vi "NMEA_Paser.vi"(8 "error in":errorcluster, 10 "INPUT":string) -> (0 "error out":errorcluster, 2 "output":string)   [LabVIEW 2015]
panel:
  # ","
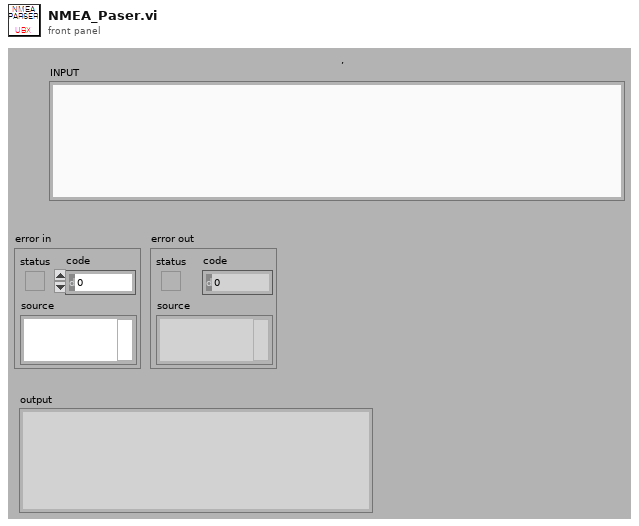
[diagram p1: front panel]
types:
  T1 = cluster{"UTC":dbl, "N/S":i8, "Latitude":dbl, "N/S 2":i8, "Longitude":dbl, "N/S 3":i8, "Speed over ground":dbl, "Course over ground":dbl}
  T2 = cluster{"UTC":dbl, "Latitude 3":dbl, "N/S":u8, "Longitude 3":dbl, "Longitude 4":dbl, "Longitude 5":dbl, "Longitude 6":dbl}
  T3 = enum16{"None", "APB", "BOD", "GGA", "GLL", "GSA", "GSV", "RMB", "RMC", "RTE", "WPL", "APA", "VTG", "XTE"}
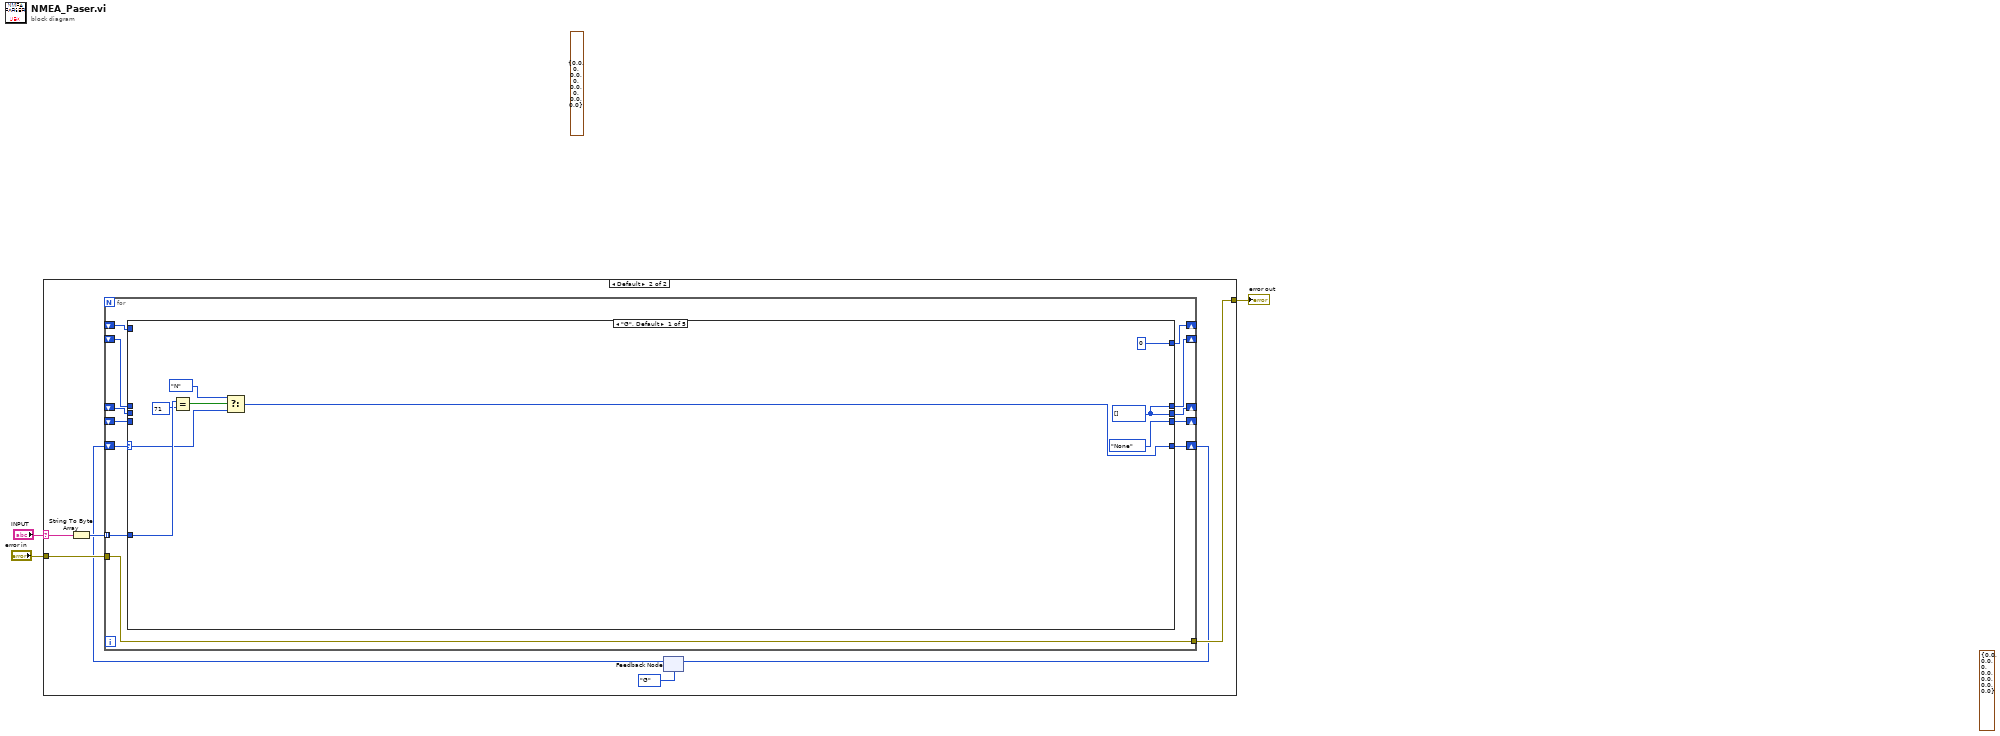
[diagram p0: block diagram]
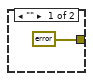
[diagram p2: hidden frame]
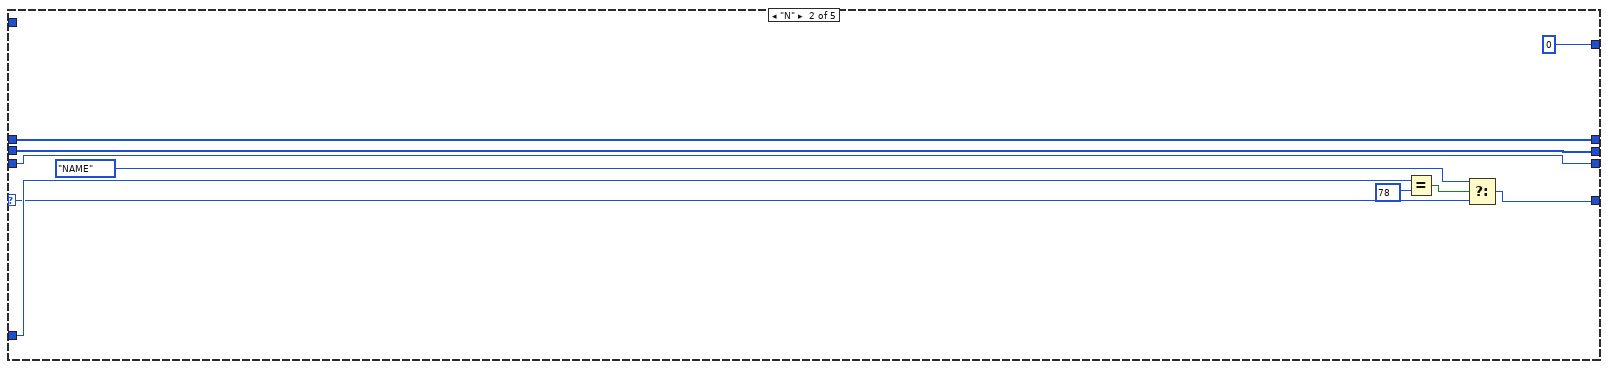
[diagram p3: hidden frame]
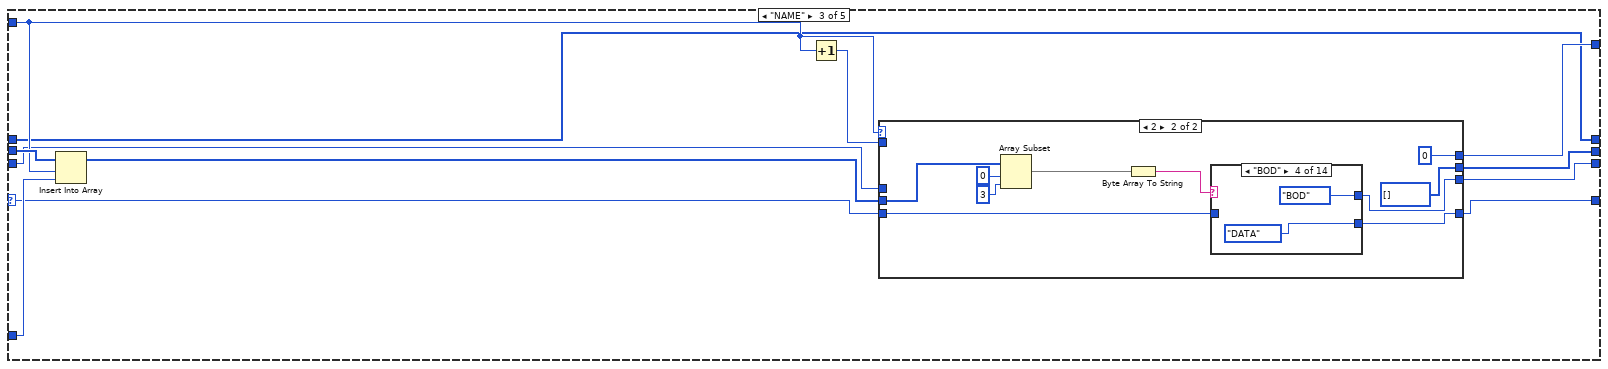
[diagram p4: hidden frame]
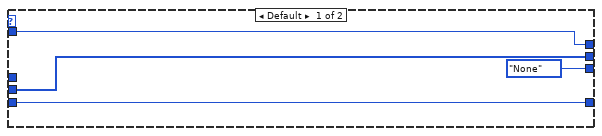
[diagram p5: hidden frame]
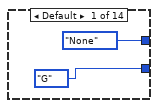
[diagram p6: hidden frame]
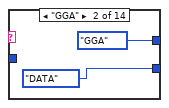
[diagram p7: hidden frame]
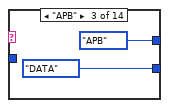
[diagram p8: hidden frame]
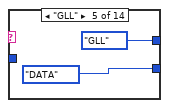
[diagram p9: hidden frame]
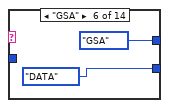
[diagram p10: hidden frame]
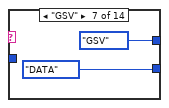
[diagram p11: hidden frame]
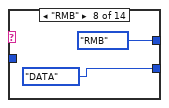
[diagram p12: hidden frame]
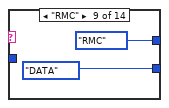
[diagram p13: hidden frame]
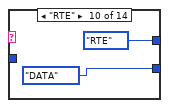
[diagram p14: hidden frame]
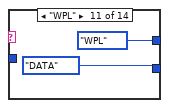
[diagram p15: hidden frame]
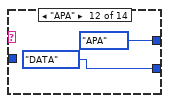
[diagram p16: hidden frame]
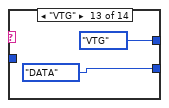
[diagram p17: hidden frame]
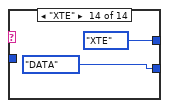
[diagram p18: hidden frame]
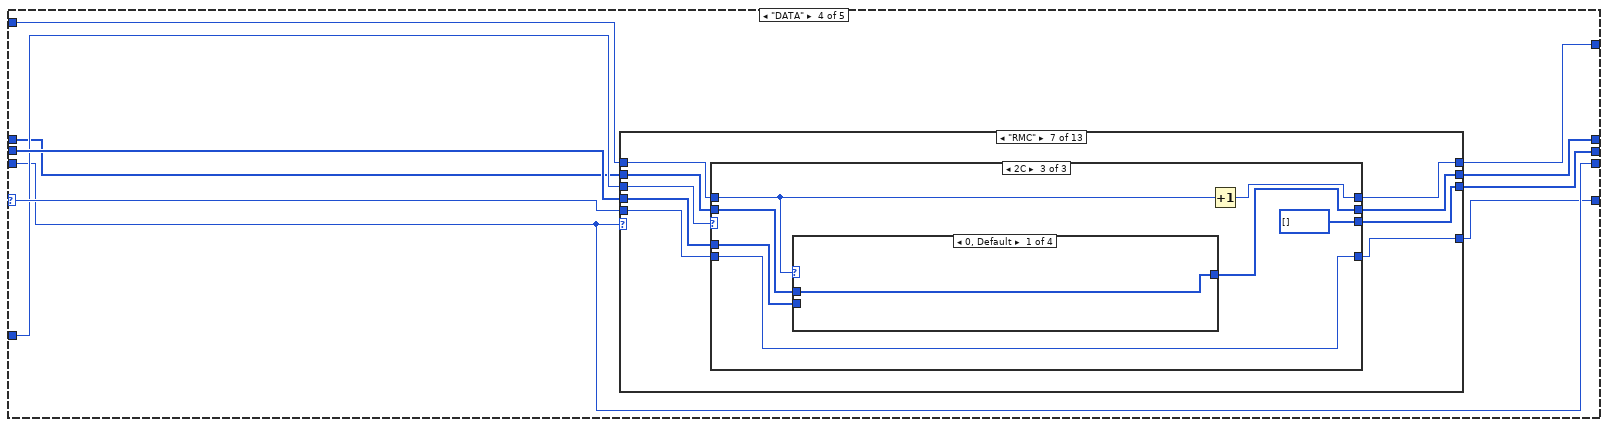
[diagram p19: hidden frame]
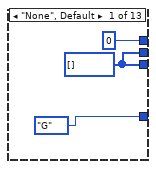
[diagram p20: hidden frame]
diagram:
  (unwired) T1 {"UTC"=0.0, "N/S"=0, "Latitude"=0.0, "N/S 2"=0, "Longitude"=0.0, "N/S 3"=0, "Speed over ground"=0.0, "Course over ground"=0.0} ("클러스터")
  (unwired) T2 {"UTC"=0.0, "Latitude 3"=0.0, "N/S"=0, "Longitude 3"=0.0, "Longitude 4"=0.0, "Longitude 5"=0.0, "Longitude 6"=0.0} ("클러스터 2")
  n1 = case shown="Default" "INPUT" {
    selector: "INPUT" -> [_ w8]
    tunnel: "error in" -> [_ w10]
    tunnel: [errorcluster {"status"=TRUE, "code"=0, "source"="Input Data is blank"} ("error in") w9] -> w2
    frame "" {
    }
    frame Default {
      n2 = String To Byte Array(string=w8) -> (unsigned byte array=w11:u8[])
      n3 = feedback #1(enum16{"G", "N", "NAME", "DATA", "END"}."G" ("t")) -> (w5:enum16{"G", "N", "NAME", "DATA", "END"})
      n4 = for {
        tunnel: w11 -> [w23] mode=indexing
        shift-right: [w22] -> _
        shift-left: _ -> [w19]
        shift-right: [w21] -> _
        shift-left: _ -> [w20]
        shift-right: [w18] -> _
        shift-left: _ -> [w17]
        shift-right: [w16] -> _
        shift-left: _ -> [w15]
        tunnel: w10 -> [w14]
        tunnel: [w14] -> w9
        shift-right: [w12] -> w6
        shift-left: w5 -> [w13]
        n5 = case shown="\"G\", Default" w13 {
          selector: w13 -> [w26 w34 w51 w105 _]
          tunnel: w23 -> [w32 w42 w53 w104 w576]
          tunnel: [0 0 w48 w99 w582] -> w22
          tunnel: [w27 w39 w44 w102 w581] -> w21
          tunnel: w20 -> [_ w39 w54 w106 w572]
          tunnel: w19 -> [_ _ w50 w101 w571]
          tunnel: [T3."None" w38 w47 w103 w583] -> w18
          tunnel: w17 -> [_ w38 w46 w103 w580]
          tunnel: [w27 w37 w45 w98 w570] -> w16
          tunnel: w15 -> [_ w37 w45 w100 w579]
          tunnel: [w24 w33 w43 w97 w569] -> w12
          frame "G", Default {
            w27 = u8[] []
            n6 = Equal?(x=w32, y=u8 71) -> (x = y?=w30:bool)
            n7 = Select(t=enum16{"G", "N", "NAME", "DATA", "END"}."N", s=w30, f=w26) -> (s? t:f=w24:enum16{"G", "N", "NAME", "DATA", "END"})
          }
          frame "N" {
            n8 = Equal?(x=w42, y=u8 78) -> (x = y?=w36:bool)
            n9 = Select(t=enum16{"G", "N", "NAME", "DATA", "END"}."NAME", s=w36, f=w34) -> (s? t:f=w33:enum16{"G", "N", "NAME", "DATA", "END"})
          }
          frame "NAME" {
            n10 = Insert Into Array(array=w54, index=w50, new element=w53) -> (w52:u8[])
            n11 = Increment(x=w50) -> (x+1=w49:i32)
            n12 = case shown="2" w50 {
              tunnel: w52 -> [w55 w61]
              tunnel: w51 -> [w58 w64]
              tunnel: [w58 w59] -> w43
              tunnel: [w57 0] -> w48
              tunnel: w49 -> [w57 _]
              tunnel: [T3."None" w62] -> w47
              tunnel: w46 -> [_ _]
              tunnel: [w55 u8[] []] -> w44
              frame Default {
              }
              frame 2 {
                n13 = Array Subset(array=w61, index=0, length=3) -> (w66:u8[])
                n14 = Byte Array To String(unsigned byte array=w66) -> (string=w65:string)
                n15 = case shown="\"BOD\"" w65 {
                  tunnel: w64 -> [_ _ _ _ _ _ _ _ _ _ _ _ _ _]
                  tunnel: [T3."None" T3."GGA" T3."APB" T3."BOD" T3."GLL" T3."GSA" T3."GSV" T3."RMB" T3."RMC" T3."RTE" T3."WPL" T3."APA" T3."VTG" T3."XTE"] -> w62
                  tunnel: [enum16{"G", "N", "NAME", "DATA", "END"}."G" ("t") enum16{"G", "N", "NAME", "DATA", "END"}."DATA" ("t") enum16{"G", "N", "NAME", "DATA", "END"}."DATA" ("t") enum16{"G", "N", "NAME", "DATA", "END"}."DATA" ("t") enum16{"G", "N", "NAME", "DATA", "END"}."DATA" ("t") enum16{"G", "N", "NAME", "DATA", "END"}."DATA" ("t") enum16{"G", "N", "NAME", "DATA", "END"}."DATA" ("t") enum16{"G", "N", "NAME", "DATA", "END"}."DATA" ("t") enum16{"G", "N", "NAME", "DATA", "END"}."DATA" ("t") enum16{"G", "N", "NAME", "DATA", "END"}."DATA" ("t") enum16{"G", "N", "NAME", "DATA", "END"}."DATA" ("t") enum16{"G", "N", "NAME", "DATA", "END"}."DATA" ("t") enum16{"G", "N", "NAME", "DATA", "END"}."DATA" ("t") enum16{"G", "N", "NAME", "DATA", "END"}."DATA" ("t")] -> w59
                  frame Default {
                  }
                  frame "GGA" {
                  }
                  frame "APB" {
                  }
                  frame "BOD" {
                  }
                  frame "GLL" {
                  }
                  frame "GSA" {
                  }
                  frame "GSV" {
                  }
                  frame "RMB" {
                  }
                  frame "RMC" {
                  }
                  frame "RTE" {
                  }
                  frame "WPL" {
                  }
                  frame "APA" {
                  }
                  frame "VTG" {
                  }
                  frame "XTE" {
                  }
                }
              }
            }
          }
          frame "DATA" {
            n16 = case shown="\"RMC\"" w103 {
              tunnel: w104 -> [_ w118 w160 w202 w238 w280 w322 w364 w400 w436 w472 w508 w541]
              tunnel: w106 -> [_ w116 w158 w200 w236 w278 w320 w362 w398 w434 w470 w506 w539]
              tunnel: w105 -> [_ w117 w159 w201 w237 w279 w321 w363 w399 w435 w471 w507 w540]
              tunnel: [w108 w115 w157 w199 w235 w277 w319 w361 w397 w433 w469 w505 w538] -> w102
              tunnel: w101 -> [_ w114 w156 w198 w234 w276 w318 w360 w396 w432 w468 w504 w537]
              tunnel: w100 -> [_ w113 w155 w197 w233 w275 w317 w359 w395 w431 w467 w503 w536]
              tunnel: [w108 w112 w154 w196 w232 w274 w316 w358 w394 w430 w466 w502 w535] -> w98
              tunnel: [0 w111 w153 w195 w231 w273 w315 w357 w393 w429 w465 w501 w534] -> w99
              tunnel: [enum16{"G", "N", "NAME", "DATA", "END"}."G" ("t") w110 w152 w194 w230 w272 w314 w356 w392 w428 w464 w500 w533] -> w97
              frame "None", Default {
                w108 = u8[] []
              }
              frame "APB" {
                n17 = case shown="Default" w118 {
                  selector: w118 -> [w123 _ _]
                  tunnel: [w121 enum16{"G", "N", "NAME", "DATA", "END"}."END" ("t") w135] -> w110
                  tunnel: w117 -> [w121 _ w135]
                  tunnel: w116 -> [w124 _ w133]
                  tunnel: [w122 u8[] [] u8[] []] -> w115
                  tunnel: w114 -> [w119 _ w129]
                  tunnel: w113 -> [w120 w126 w132]
                  tunnel: [w120 w126 w131] -> w112
                  tunnel: [w119 0 w130] -> w111
                  frame Default {
                    n18 = Insert Into Array(array=w124, new element=w123) -> (w122:u8[])  [unwired: 1 in]
                  }
                  frame 42 {
                  }
                  frame 44 {
                    n19 = case shown="1, 2, 4..7, 9, 10, 12, 14" w129 {
                      tunnel: w133 -> [_ w138 w141 w149]
                      tunnel: w132 -> [w136 w139 w145 w147]
                      tunnel: [w136 w137 w144 w151] -> w131
                      frame 0, Default {
                      }
                      frame 1, 2, 4..7, 9, 10, 12, 14 {
                        n20 = Insert Into Array(array=w139, new element=w138) -> (w137:u8[])  [unwired: 1 in]
                      }
                      frame 3 {
                        n21 = Byte Array To String(unsigned byte array=w141) -> (string=w143:string)
                        n22 = Fract/Exp String To Number(string=w143) -> (number=w142:dbl)  [unwired: 3 in, 1 out]
                        n23 = Type Cast(type=w141, x=w142) -> (*(type *) &x=w140:u8[])
                        n24 = Insert Into Array(array=w145, new element=w140) -> (w144:u8[])  [unwired: 1 in]
                      }
                      frame 8, 11 {
                        n25 = Byte Array To String(unsigned byte array=w149) -> (string=w150:string)
                        n26 = Decimal String To Number(string=w150) -> (number=w148:i32)  [unwired: 2 in, 1 out]
                        n27 = Type Cast(type=w147, x=w148) -> (*(type *) &x=w146:u8[])
                        n28 = Insert Into Array(array=w147, new element=w146) -> (w151:u8[])  [unwired: 1 in]
                      }
                    }
                    n29 = Increment(x=w129) -> (x+1=w130:i32)
                  }
                }
              }
              frame "GGA" {
                n30 = case shown="2C" w160 {
                  selector: w160 -> [w165 _ _]
                  tunnel: [w163 enum16{"G", "N", "NAME", "DATA", "END"}."END" ("t") w177] -> w152
                  tunnel: w159 -> [w163 _ w177]
                  tunnel: w158 -> [w166 _ w171]
                  tunnel: [w164 u8[] [] u8[] []] -> w157
                  tunnel: w156 -> [w161 _ w173]
                  tunnel: w155 -> [w162 w168 w172]
                  tunnel: [w162 w168 w175] -> w154
                  tunnel: [w161 0 w174] -> w153
                  frame Default {
                    n31 = Insert Into Array(array=w166, new element=w165) -> (w164:u8[])  [unwired: 1 in]
                  }
                  frame 42 {
                  }
                  frame 44 {
                    n32 = case shown="3, 5, 10, 12" w173 {
                      tunnel: w171 -> [_ w179 w183 w191]
                      tunnel: w172 -> [w178 w181 w185 w189]
                      tunnel: [w178 w180 w187 w193] -> w175
                      frame 0, Default {
                      }
                      frame 3, 5, 10, 12 {
                        n33 = Insert Into Array(array=w181, new element=w179) -> (w180:u8[])  [unwired: 1 in]
                      }
                      frame 1, 2, 4, 8, 9, 11, 13 {
                        n34 = Byte Array To String(unsigned byte array=w183) -> (string=w186:string)
                        n35 = Fract/Exp String To Number(string=w186) -> (number=w184:dbl)  [unwired: 3 in, 1 out]
                        n36 = Type Cast(type=w183, x=w184) -> (*(type *) &x=w182:u8[])
                        n37 = Insert Into Array(array=w185, new element=w182) -> (w187:u8[])  [unwired: 1 in]
                      }
                      frame 6, 7 {
                        n38 = Byte Array To String(unsigned byte array=w191) -> (string=w192:string)
                        n39 = Decimal String To Number(string=w192) -> (number=w190:i32)  [unwired: 2 in, 1 out]
                        n40 = Type Cast(type=w189, x=w190) -> (*(type *) &x=w188:u8[])
                        n41 = Insert Into Array(array=w189, new element=w188) -> (w193:u8[])  [unwired: 1 in]
                      }
                    }
                    n42 = Increment(x=w173) -> (x+1=w174:i32)
                  }
                }
              }
              frame "GLL" {
                n43 = case shown="Default" w202 {
                  selector: w202 -> [w207 _ _]
                  tunnel: [w205 enum16{"G", "N", "NAME", "DATA", "END"}."END" ("t") w219] -> w194
                  tunnel: w201 -> [w205 _ w219]
                  tunnel: w200 -> [w208 _ w217]
                  tunnel: [w206 u8[] [] u8[] []] -> w199
                  tunnel: w198 -> [w203 _ w213]
                  tunnel: w197 -> [w204 w210 w216]
                  tunnel: [w204 w210 w215] -> w196
                  tunnel: [w203 0 w214] -> w195
                  frame Default {
                    n44 = Insert Into Array(array=w208, new element=w207) -> (w206:u8[])  [unwired: 1 in]
                  }
                  frame 42 {
                  }
                  frame 44 {
                    n45 = case shown="0, Default" w213 {
                      tunnel: w217 -> [_ w222 w225]
                      tunnel: w216 -> [w220 w223 w229]
                      tunnel: [w220 w221 w228] -> w215
                      frame 0, Default {
                      }
                      frame 2, 4, 6 {
                        n46 = Insert Into Array(array=w223, new element=w222) -> (w221:u8[])  [unwired: 1 in]
                      }
                      frame 1, 3, 5 {
                        n47 = Byte Array To String(unsigned byte array=w225) -> (string=w227:string)
                        n48 = Fract/Exp String To Number(string=w227) -> (number=w226:dbl)  [unwired: 3 in, 1 out]
                        n49 = Type Cast(type=w225, x=w226) -> (*(type *) &x=w224:u8[])
                        n50 = Insert Into Array(array=w229, new element=w224) -> (w228:u8[])  [unwired: 1 in]
                      }
                    }
                    n51 = Increment(x=w213) -> (x+1=w214:i32)
                  }
                }
              }
              frame "GSA" {
                n52 = case shown="2A" w238 {
                  selector: w238 -> [w243 _ _]
                  tunnel: [w241 enum16{"G", "N", "NAME", "DATA", "END"}."END" ("t") w255] -> w230
                  tunnel: w237 -> [w241 _ w255]
                  tunnel: w236 -> [w244 _ w253]
                  tunnel: [w242 u8[] [] u8[] []] -> w235
                  tunnel: w234 -> [w239 _ w249]
                  tunnel: w233 -> [w240 w246 w252]
                  tunnel: [w240 w246 w251] -> w232
                  tunnel: [w239 0 w250] -> w231
                  frame Default {
                    n53 = Insert Into Array(array=w244, new element=w243) -> (w242:u8[])  [unwired: 1 in]
                  }
                  frame 42 {
                  }
                  frame 44 {
                    n54 = case shown="3..14" w249 {
                      tunnel: w253 -> [_ w257 w261 w269]
                      tunnel: w252 -> [w256 w258 w265 w267]
                      tunnel: [w256 w259 w264 w271] -> w251
                      frame 0, Default {
                      }
                      frame 1 {
                        n55 = Insert Into Array(array=w258, new element=w257) -> (w259:u8[])  [unwired: 1 in]
                      }
                      frame 15..17 {
                        n56 = Byte Array To String(unsigned byte array=w261) -> (string=w263:string)
                        n57 = Fract/Exp String To Number(string=w263) -> (number=w262:dbl)  [unwired: 3 in, 1 out]
                        n58 = Type Cast(type=w261, x=w262) -> (*(type *) &x=w260:u8[])
                        n59 = Insert Into Array(array=w265, new element=w260) -> (w264:u8[])  [unwired: 1 in]
                      }
                      frame 3..14 {
                        n60 = Byte Array To String(unsigned byte array=w269) -> (string=w270:string)
                        n61 = Decimal String To Number(string=w270) -> (number=w266:i32)  [unwired: 2 in, 1 out]
                        n62 = Type Cast(type=w267, x=w266) -> (*(type *) &x=w268:u8[])
                        n63 = Insert Into Array(array=w267, new element=w268) -> (w271:u8[])  [unwired: 1 in]
                      }
                    }
                    n64 = Increment(x=w249) -> (x+1=w250:i32)
                  }
                }
              }
              frame "RMB" {
                n65 = case shown="2A" w280 {
                  selector: w280 -> [w285 _ _]
                  tunnel: [w283 enum16{"G", "N", "NAME", "DATA", "END"}."END" ("t") w297] -> w272
                  tunnel: w279 -> [w283 _ w297]
                  tunnel: w278 -> [w286 _ w295]
                  tunnel: [w284 u8[] [] u8[] []] -> w277
                  tunnel: w276 -> [w281 _ w291]
                  tunnel: w275 -> [w282 w288 w294]
                  tunnel: [w282 w288 w293] -> w274
                  tunnel: [w281 0 w292] -> w273
                  frame Default {
                    n66 = Insert Into Array(array=w286, new element=w285) -> (w284:u8[])  [unwired: 1 in]
                  }
                  frame 42 {
                  }
                  frame 44 {
                    n67 = case shown="0, Default" w291 {
                      tunnel: w295 -> [_ w300 w303 w311]
                      tunnel: w294 -> [w298 w301 w307 w309]
                      tunnel: [w298 w299 w306 w313] -> w293
                      frame 0, Default {
                      }
                      frame 1, 3, 7, 9, 13 {
                        n68 = Insert Into Array(array=w301, new element=w300) -> (w299:u8[])  [unwired: 1 in]
                      }
                      frame 2, 6, 8, 10..12 {
                        n69 = Byte Array To String(unsigned byte array=w303) -> (string=w305:string)
                        n70 = Fract/Exp String To Number(string=w305) -> (number=w304:dbl)  [unwired: 3 in, 1 out]
                        n71 = Type Cast(type=w303, x=w304) -> (*(type *) &x=w302:u8[])
                        n72 = Insert Into Array(array=w307, new element=w302) -> (w306:u8[])  [unwired: 1 in]
                      }
                      frame 4, 5 {
                        n73 = Byte Array To String(unsigned byte array=w311) -> (string=w312:string)
                        n74 = Decimal String To Number(string=w312) -> (number=w308:i32)  [unwired: 2 in, 1 out]
                        n75 = Type Cast(type=w309, x=w308) -> (*(type *) &x=w310:u8[])
                        n76 = Insert Into Array(array=w309, new element=w310) -> (w313:u8[])  [unwired: 1 in]
                      }
                    }
                    n77 = Increment(x=w291) -> (x+1=w292:i32)
                  }
                }
              }
              frame "RMC" {
                n78 = case shown="2C" w322 {
                  selector: w322 -> [w327 _ _]
                  tunnel: [w325 enum16{"G", "N", "NAME", "DATA", "END"}."END" ("t") w339] -> w314
                  tunnel: w321 -> [w325 _ w339]
                  tunnel: w320 -> [w328 _ w337]
                  tunnel: [w326 u8[] [] u8[] []] -> w319
                  tunnel: w318 -> [w323 _ w333]
                  tunnel: w317 -> [w324 w330 w336]
                  tunnel: [w324 w330 w335] -> w316
                  tunnel: [w323 0 w334] -> w315
                  frame Default {
                    n79 = Insert Into Array(array=w328, new element=w327) -> (w326:u8[])  [unwired: 1 in]
                  }
                  frame 42 {
                  }
                  frame 44 {
                    n80 = case shown="0, Default" w333 {
                      tunnel: w337 -> [_ w342 w345 w353]
                      tunnel: w336 -> [w340 w343 w349 w351]
                      tunnel: [w340 w341 w348 w355] -> w335
                      frame 0, Default {
                      }
                      frame 2, 4, 6, 11 {
                        n81 = Insert Into Array(array=w343, new element=w342) -> (w341:u8[])  [unwired: 1 in]
                      }
                      frame 1, 3, 5, 7, 8, 10 {
                        n82 = Byte Array To String(unsigned byte array=w345) -> (string=w347:string)
                        n83 = Fract/Exp String To Number(string=w347) -> (number=w346:dbl)  [unwired: 3 in, 1 out]
                        n84 = Type Cast(type=w345, x=w346) -> (*(type *) &x=w344:u8[])
                        n85 = Insert Into Array(array=w349, new element=w344) -> (w348:u8[])  [unwired: 1 in]
                      }
                      frame 9 {
                        n86 = Byte Array To String(unsigned byte array=w353) -> (string=w354:string)
                        n87 = Decimal String To Number(string=w354) -> (number=w350:i32)  [unwired: 2 in, 1 out]
                        n88 = Type Cast(type=w351, x=w350) -> (*(type *) &x=w352:u8[])
                        n89 = Insert Into Array(array=w351, new element=w352) -> (w355:u8[])  [unwired: 1 in]
                      }
                    }
                    n90 = Increment(x=w333) -> (x+1=w334:i32)
                  }
                }
              }
              frame "XTE" {
                n91 = case shown="2A" w364 {
                  selector: w364 -> [w369 _ _]
                  tunnel: [w367 enum16{"G", "N", "NAME", "DATA", "END"}."END" ("t") w381] -> w356
                  tunnel: w363 -> [w367 _ w381]
                  tunnel: w362 -> [w370 _ w379]
                  tunnel: [w368 u8[] [] u8[] []] -> w361
                  tunnel: w360 -> [w365 _ w375]
                  tunnel: w359 -> [w366 w372 w378]
                  tunnel: [w366 w372 w377] -> w358
                  tunnel: [w365 0 w376] -> w357
                  frame Default {
                    n92 = Insert Into Array(array=w370, new element=w369) -> (w368:u8[])  [unwired: 1 in]
                  }
                  frame 42 {
                  }
                  frame 44 {
                    n93 = case shown="1, 2, 4, 5" w375 {
                      tunnel: w379 -> [_ w384 w387]
                      tunnel: w378 -> [w382 w385 w391]
                      tunnel: [w382 w383 w390] -> w377
                      frame 0, Default {
                      }
                      frame 1, 2, 4, 5 {
                        n94 = Insert Into Array(array=w385, new element=w384) -> (w383:u8[])  [unwired: 1 in]
                      }
                      frame 3 {
                        n95 = Byte Array To String(unsigned byte array=w387) -> (string=w389:string)
                        n96 = Fract/Exp String To Number(string=w389) -> (number=w388:dbl)  [unwired: 3 in, 1 out]
                        n97 = Type Cast(type=w387, x=w388) -> (*(type *) &x=w386:u8[])
                        n98 = Insert Into Array(array=w391, new element=w386) -> (w390:u8[])  [unwired: 1 in]
                      }
                    }
                    n99 = Increment(x=w375) -> (x+1=w376:i32)
                  }
                }
              }
              frame "VTG" {
                n100 = case shown="Default" w400 {
                  selector: w400 -> [w405 _ _]
                  tunnel: [w403 enum16{"G", "N", "NAME", "DATA", "END"}."END" ("t") w417] -> w392
                  tunnel: w399 -> [w403 _ w417]
                  tunnel: w398 -> [w406 _ w415]
                  tunnel: [w404 u8[] [] u8[] []] -> w397
                  tunnel: w396 -> [w401 _ w411]
                  tunnel: w395 -> [w402 w408 w414]
                  tunnel: [w402 w408 w413] -> w394
                  tunnel: [w401 0 w412] -> w393
                  frame Default {
                    n101 = Insert Into Array(array=w406, new element=w405) -> (w404:u8[])  [unwired: 1 in]
                  }
                  frame 42 {
                  }
                  frame 44 {
                    n102 = case shown="2, 4, 6, 8" w411 {
                      tunnel: w415 -> [_ w420 w423]
                      tunnel: w414 -> [w418 w421 w427]
                      tunnel: [w418 w419 w426] -> w413
                      frame 0, Default {
                      }
                      frame 2, 4, 6, 8 {
                        n103 = Insert Into Array(array=w421, new element=w420) -> (w419:u8[])  [unwired: 1 in]
                      }
                      frame 1, 3, 5, 7 {
                        n104 = Byte Array To String(unsigned byte array=w423) -> (string=w425:string)
                        n105 = Fract/Exp String To Number(string=w425) -> (number=w424:dbl)  [unwired: 3 in, 1 out]
                        n106 = Type Cast(type=w423, x=w424) -> (*(type *) &x=w422:u8[])
                        n107 = Insert Into Array(array=w427, new element=w422) -> (w426:u8[])  [unwired: 1 in]
                      }
                    }
                    n108 = Increment(x=w411) -> (x+1=w412:i32)
                  }
                }
              }
              frame "WPL" {
                n109 = case shown="2C" w436 {
                  selector: w436 -> [w441 _ _]
                  tunnel: [w439 enum16{"G", "N", "NAME", "DATA", "END"}."END" ("t") w453] -> w428
                  tunnel: w435 -> [w439 _ w453]
                  tunnel: w434 -> [w442 _ w451]
                  tunnel: [w440 u8[] [] u8[] []] -> w433
                  tunnel: w432 -> [w437 _ w447]
                  tunnel: w431 -> [w438 w444 w450]
                  tunnel: [w438 w444 w449] -> w430
                  tunnel: [w437 0 w448] -> w429
                  frame Default {
                    n110 = Insert Into Array(array=w442, new element=w441) -> (w440:u8[])  [unwired: 1 in]
                  }
                  frame 42 {
                  }
                  frame 44 {
                    n111 = case shown="2, 4, 5" w447 {
                      tunnel: w451 -> [_ w456 w459]
                      tunnel: w450 -> [w454 w457 w463]
                      tunnel: [w454 w455 w462] -> w449
                      frame 0, Default {
                      }
                      frame 2, 4, 5 {
                        n112 = Insert Into Array(array=w457, new element=w456) -> (w455:u8[])  [unwired: 1 in]
                      }
                      frame 1, 3 {
                        n113 = Byte Array To String(unsigned byte array=w459) -> (string=w461:string)
                        n114 = Fract/Exp String To Number(string=w461) -> (number=w460:dbl)  [unwired: 3 in, 1 out]
                        n115 = Type Cast(type=w459, x=w460) -> (*(type *) &x=w458:u8[])
                        n116 = Insert Into Array(array=w463, new element=w458) -> (w462:u8[])  [unwired: 1 in]
                      }
                    }
                    n117 = Increment(x=w447) -> (x+1=w448:i32)
                  }
                }
              }
              frame "RTE" {
                n118 = case shown="2A" w472 {
                  selector: w472 -> [w477 _ _]
                  tunnel: [w475 enum16{"G", "N", "NAME", "DATA", "END"}."END" ("t") w489] -> w464
                  tunnel: w471 -> [w475 _ w489]
                  tunnel: w470 -> [w478 _ w487]
                  tunnel: [w476 u8[] [] u8[] []] -> w469
                  tunnel: w468 -> [w473 _ w483]
                  tunnel: w467 -> [w474 w480 w486]
                  tunnel: [w474 w480 w485] -> w466
                  tunnel: [w473 0 w484] -> w465
                  frame Default {
                    n119 = Insert Into Array(array=w478, new element=w477) -> (w476:u8[])  [unwired: 1 in]
                  }
                  frame 42 {
                  }
                  frame 44 {
                    n120 = case shown="1, 2, 4" w483 {
                      tunnel: w487 -> [_ w492 w497]
                      tunnel: w486 -> [w490 w493 w495]
                      tunnel: [w490 w491 w499] -> w485
                      frame 0 {
                      }
                      frame 3, 5, Default {
                        n121 = Insert Into Array(array=w493, new element=w492) -> (w491:u8[])  [unwired: 1 in]
                      }
                      frame 1, 2, 4 {
                        n122 = Byte Array To String(unsigned byte array=w497) -> (string=w498:string)
                        n123 = Decimal String To Number(string=w498) -> (number=w494:i32)  [unwired: 2 in, 1 out]
                        n124 = Type Cast(type=w495, x=w494) -> (*(type *) &x=w496:u8[])
                        n125 = Insert Into Array(array=w495, new element=w496) -> (w499:u8[])  [unwired: 1 in]
                      }
                    }
                    n126 = Increment(x=w483) -> (x+1=w484:i32)
                  }
                }
              }
              frame "GSV" {
                n127 = case shown="2C" w508 {
                  selector: w508 -> [w513 _ _]
                  tunnel: [w511 enum16{"G", "N", "NAME", "DATA", "END"}."END" ("t") w525] -> w500
                  tunnel: w507 -> [w511 _ w525]
                  tunnel: w506 -> [w514 _ w523]
                  tunnel: [w512 u8[] [] u8[] []] -> w505
                  tunnel: w504 -> [w509 _ w519]
                  tunnel: w503 -> [w510 w516 w522]
                  tunnel: [w510 w516 w521] -> w502
                  tunnel: [w509 0 w520] -> w501
                  frame Default {
                    n128 = Insert Into Array(array=w514, new element=w513) -> (w512:u8[])  [unwired: 1 in]
                  }
                  frame 42 {
                  }
                  frame 44 {
                    n129 = case shown="Default" w519 {
                      tunnel: w523 -> [w529 _]
                      tunnel: w522 -> [w527 w532]
                      tunnel: [w531 w532] -> w521
                      frame Default {
                        n130 = Byte Array To String(unsigned byte array=w529) -> (string=w530:string)
                        n131 = Decimal String To Number(string=w530) -> (number=w526:i32)  [unwired: 2 in, 1 out]
                        n132 = Type Cast(type=w527, x=w526) -> (*(type *) &x=w528:u8[])
                        n133 = Insert Into Array(array=w527, new element=w528) -> (w531:u8[])  [unwired: 1 in]
                      }
                      frame 0 {
                      }
                    }
                    n134 = Increment(x=w519) -> (x+1=w520:i32)
                  }
                }
              }
              frame "BOD" {
                n135 = case shown="2A" w541 {
                  selector: w541 -> [w546 _ _]
                  tunnel: [w544 enum16{"G", "N", "NAME", "DATA", "END"}."END" ("t") w558] -> w533
                  tunnel: w540 -> [w544 _ w558]
                  tunnel: w539 -> [w547 _ w556]
                  tunnel: [w545 u8[] [] u8[] []] -> w538
                  tunnel: w537 -> [w542 _ w552]
                  tunnel: w536 -> [w543 w549 w555]
                  tunnel: [w543 w549 w554] -> w535
                  tunnel: [w542 0 w553] -> w534
                  frame Default {
                    n136 = Insert Into Array(array=w547, new element=w546) -> (w545:u8[])  [unwired: 1 in]
                  }
                  frame 42 {
                  }
                  frame 44 {
                    n137 = case shown="0, Default" w552 {
                      tunnel: w556 -> [_ w561 w564]
                      tunnel: w555 -> [w559 w562 w568]
                      tunnel: [w559 w560 w567] -> w554
                      frame 0, Default {
                      }
                      frame 2, 4..6 {
                        n138 = Insert Into Array(array=w562, new element=w561) -> (w560:u8[])  [unwired: 1 in]
                      }
                      frame 1, 3 {
                        n139 = Byte Array To String(unsigned byte array=w564) -> (string=w566:string)
                        n140 = Fract/Exp String To Number(string=w566) -> (number=w565:dbl)  [unwired: 3 in, 1 out]
                        n141 = Type Cast(type=w564, x=w565) -> (*(type *) &x=w563:u8[])
                        n142 = Insert Into Array(array=w568, new element=w563) -> (w567:u8[])  [unwired: 1 in]
                      }
                    }
                    n143 = Increment(x=w552) -> (x+1=w553:i32)
                  }
                }
              }
            }
          }
          frame "END" {
            n144 = Equal?(x=w576, y=u8 10) -> (x = y?=w575:bool)
            n145 = Equal?(x=w576, y=u8 13) -> (x = y?=w574:bool)
            n146 = Or(x=w575, y=w574) -> (x .or. y?=w573:bool)
            n147 = case shown="False" w573 {
              tunnel: [w588 T3."None"] -> w583
              tunnel: [w586 0] -> w582
              tunnel: [w587 w591] -> w581
              tunnel: w580 -> [w588 w596]
              tunnel: w579 -> [w585 w592]
              tunnel: w572 -> [w587 _]
              tunnel: w571 -> [w586 _]
              tunnel: [w585 w591] -> w570
              tunnel: [enum16{"G", "N", "NAME", "DATA", "END"}."END" ("t") enum16{"G", "N", "NAME", "DATA", "END"}."G" ("t")] -> w569
              frame False {
              }
              frame True {
                w591 = u8[] []
                n148 = case shown="\"GGA\"" w596 {
                  tunnel: [_ u8[] [65, 80, 66] u8[] [66, 79, 68] u8[] [71, 71, 65] u8[] [71, 76, 76] u8[] [71, 83, 65] u8[] [71, 83, 86] u8[] [82, 77, 66] u8[] [82, 77, 67] u8[] [82, 84, 69] u8[] [87, 80, 76] u8[] [86, 84, 71] u8[] [88, 84, 69]] -> w594
                  frame "None", Default {
                  }
                  frame "APB" {
                  }
                  frame "BOD" {
                  }
                  frame "GGA" {
                  }
                  frame "GLL" {
                  }
                  frame "GSA" {
                  }
                  frame "GSV" {
                  }
                  frame "RMB" {
                  }
                  frame "RMC" {
                  }
                  frame "RTE" {
                  }
                  frame "WPL" {
                  }
                  frame "VTG" {
                  }
                  frame "XTE" {
                  }
                }
                n149 = Insert Into Array(array=w592, index=0, new element=w594) -> (w593:u8[])
                n150 = Byte Array To String(unsigned byte array=w593) -> (string=→"output":string)
              }
            }
          }
        }
      }
      n151 = feedback-in #1(w6) -> ()
    }
  }
  "error out" <- w2
